vi "CreateCSV.vi"() -> ()   [LabVIEW 2018]
panel:
  out "String":string
  out "Boolean 2":bool
  in  "OK Button":bool
  out "Boolean":bool
  out "Output Text":string
  out "Next Datum":string
  in  "Save File":bool
  in  "Save File Path":string
  in  "Pressure 2":dbl
  in  "Pressure 1":dbl
  in  "Temperature 2":dbl
  in  "Temperature 1":dbl
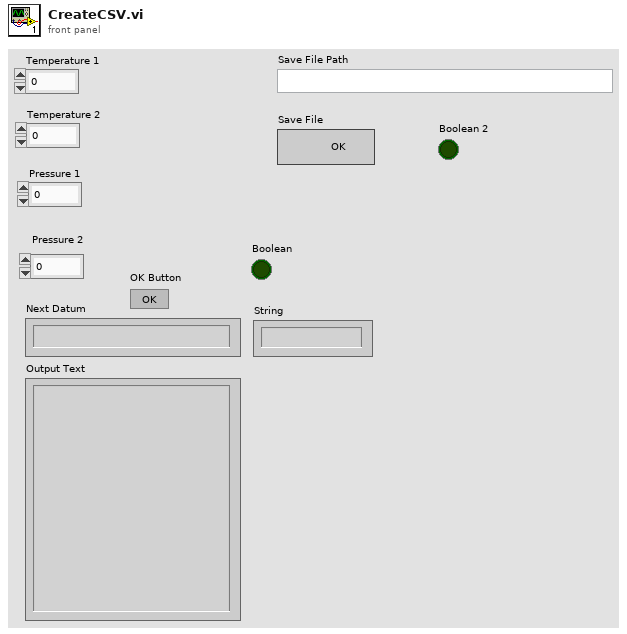
[diagram p1: front panel]
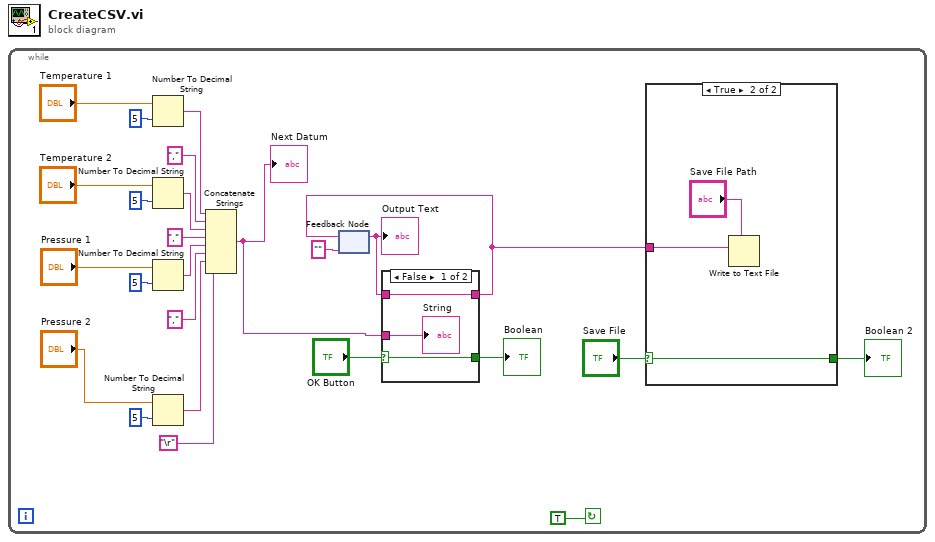
[diagram p0: block diagram]
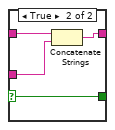
[diagram p3: hidden frame]
diagram:
  n1 = while {
    stop <- TRUE continue-if-true
    n2 = Number To Decimal String(number="Temperature 1", width (-)=5) -> (decimal integer string=w16:string)
    n3 = Number To Decimal String(number="Temperature 2", width (-)=5) -> (decimal integer string=w14:string)
    n4 = Number To Decimal String(number="Pressure 1", width (-)=5) -> (decimal integer string=w12:string)
    n5 = Number To Decimal String(number="Pressure 2", width (-)=5) -> (decimal integer string=w10:string)
    n6 = Concatenate Strings(w16, ",", w14, ",", w12, ",", w10, "\r") -> (w8:string)
    "Next Datum" <- w8
    n7 = feedback #1("") -> (w4:string)
    "Output Text" <- w4
    n8 = case shown="False" "OK Button" {
      selector: "OK Button" -> [w32 w36]
      tunnel: w8 -> [w30 w35]
      tunnel: [w32 w36] -> w7
      tunnel: [w31 w34] -> w1
      tunnel: w4 -> [w31 w33]
      frame False {
        "String" <- w30
      }
      frame True {
        n9 = Concatenate Strings(w33, w35) -> (w34:string)
      }
    }
    "Boolean" <- w7
    n10 = feedback-in #1(w1) -> ()
    n11 = case shown="True" "Save File" {
      selector: "Save File" -> [w26 w29]
      tunnel: [w26 w29] -> w2
      tunnel: w1 -> [_ w28]
      frame False {
      }
      frame True {
        n12 = Write to Text File(prompt (Choose or enter file path)="Save File Path", text=w28) -> ()  [unwired: 2 in, 3 out]
      }
    }
    "Boolean 2" <- w2
  }
